vi "Set context rings.vi"(0 "Display State In":T1, 5 "Column":i32, 7 "Strings":cluster{"Strings":string[]}[][](array[cluster]), 9 "Container State":T6, 11 "error in (no error)":errorcluster) -> (4 "Display State Out":T1, 15 "error out":errorcluster)   [LabVIEW 2015, in "KTable.xctl"]
uses:
  KTable.xctl
  <vilib>/_xctls/Container State.ctl
  State.ctl
  ColumnSpec.ctl
  ColumnType.ctl
  Table Properties.ctl
  Events.ctl
  Event Data.ctl
  Event Type.ctl
  <vilib>/_xctls/XControlSupport.lvlib
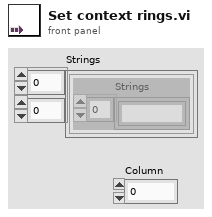
[diagram p1: front panel]
types:
  T1 = typedef "KTable.xctl/State.ctl" = cluster{"Columns":T2[], "Listbox":refnum<vi>, "Default row":string[], "Properties":T4, "Events":T5, "Locked":bool[][], "Size":cluster{"Rows":i32, "Columns":i32}, "rings":i32[][], "DefColors":u32[]}
  T2 = typedef "KTable.xctl/ColumnSpec.ctl" = cluster{"Name":string, "Type":T3, "Width":i32, "Strings":string[], "Position":enum16{"Left", "Center", "Right"}, "locked":bool, "cds":cluster{"Strings":string[]}[][]}
  T3 = typedef "KTable.xctl/ColumnType.ctl" = enum16{"String", "Enum", "Int", "Double", "Boolean", "Ring", "Formula", "Color"}
  T4 = typedef "KTable.xctl/Table Properties.ctl" = cluster{"Vertical scrollbar":bool, "User add/delete":bool, "Max rows":i32, "Row headers":bool}
  T5 = typedef "KTable.xctl/Events.ctl" = cluster{"Items Changed":refnum<user-event>}
  T6 = typedef "XControlSupport.lvlib/Container State.ctl" = cluster{"Indicator?":bool, "Run Mode?":bool, " Refnum":refnum<vi>}
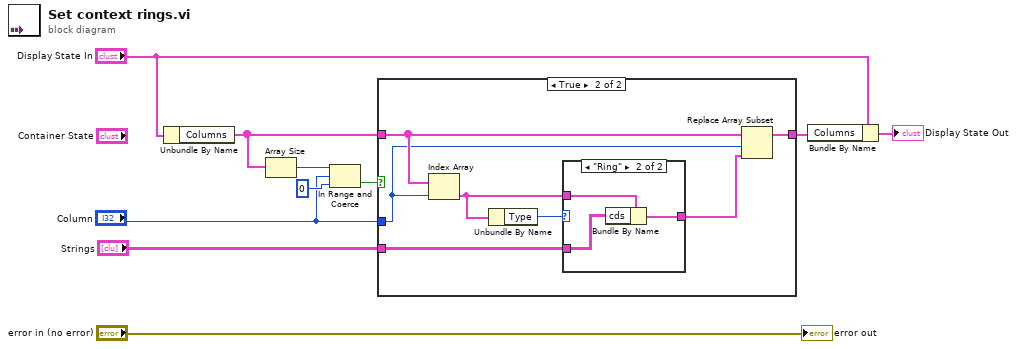
[diagram p0: block diagram]
diagram:
  n1 = Unbundle By Name("Display State In") -> ("Columns"=w6:T2[])
  n2 = Array Size(array=w6) -> (size(s)=w9:i32)
  n3 = In Range and Coerce(upper limit=w9, x="Column", lower limit=0) -> (In Range?=w7:bool)  [unwired: 1 out]
  n4 = case shown="True" w7 {
    tunnel: "Column" -> [_ w14]
    tunnel: w6 -> [w11 w15]
    tunnel: "Strings" -> [_ w16]
    tunnel: [w11 w12] -> w5
    frame False {
    }
    frame True {
      n5 = Index Array(array=w15, index=w14) -> (element=w17:T2)
      n6 = Unbundle By Name(w17) -> ("Type"=w18:T3)
      n7 = case shown="\"Ring\"" w18 {
        tunnel: w17 -> [w19 w22]
        tunnel: w16 -> [_ w21]
        tunnel: [w19 w20] -> w13
        frame "String", Default {
        }
        frame "Ring" {
          n8 = Bundle By Name(cluster=w22, "cds"=w21) -> (w20:T2)
        }
      }
      n9 = Replace Array Subset(array=w15, new element=w13, index=w14) -> (w12:T2[])
    }
  }
  n10 = Bundle By Name(cluster="Display State In", "Columns"=w5) -> (→"Display State Out":T1)
  "error out" <- "error in (no error)"
